vi "Format Date to SQL.vi"(1 "Date":timestamp) -> (0 "SQL Date":string)   [LabVIEW 2018, in "Transaction.lvclass"]
uses:
  Transaction.lvclass
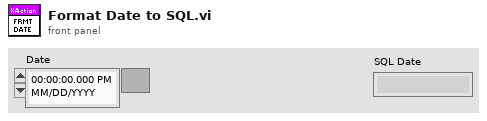
[diagram p1: front panel]
types:
  T1 = typedef "LVDateTimeRec.ctl" = cluster{"fractional second":dbl, "second":i32, "minute":i32, "hour":i32, "day of month":i32, "month":i32, "year":i32, "day of week":i32, "day of year":i32, "DST":i32}
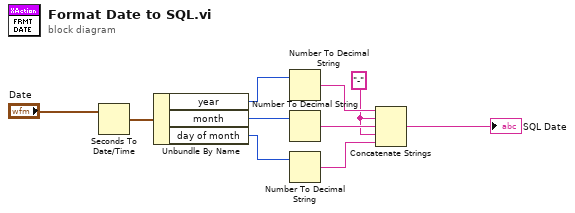
[diagram p0: block diagram]
diagram:
  w6 = "-"
  n1 = Seconds To Date/Time(time stamp (now)="Date") -> (date time rec=w2:T1)  [unwired: 1 in]
  n2 = Unbundle By Name(w2) -> ("year"=w3:i32, "month"=w4:i32, "day of month"=w5:i32)
  n3 = Number To Decimal String(number=w3) -> (decimal integer string=w7:string)  [unwired: 1 in]
  n4 = Number To Decimal String(number=w4) -> (decimal integer string=w8:string)  [unwired: 1 in]
  n5 = Number To Decimal String(number=w5) -> (decimal integer string=w9:string)  [unwired: 1 in]
  n6 = Concatenate Strings(w7, w6, w8, w6, w9) -> (→"SQL Date":string)
